vi "Goal Angle Calculation.vi"(5 "Target-Goal X Translation(trans)":dbl, 7 "Target Distance (v)":dbl, 11 "Field-Rel Tgt Angle (theta)":dbl format="%#_13g") -> (1 "Goal Distance (r)":dbl, 3 "Goal Angle (phi)":dbl)   [LabVIEW 2013]
panel:
  out "Vis Tgt - Perp Point Distance (dv)":dbl
  out "Perp. Distance (h)":dbl
  out "Goal - Perp Point Distance (dg)":dbl
  # "d = dg + dv"
  # "goal"
  # "vision target"
  # "dg"
  # "dv"
  # "h"
  # "v"
  # "r"
  # "theta"
  # "phi"
  # "cam angle + servo angle + gyro angle"
  # "robot"
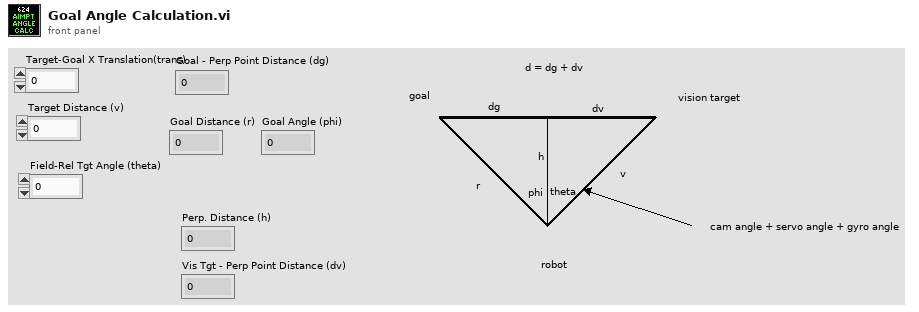
[diagram p1: front panel]
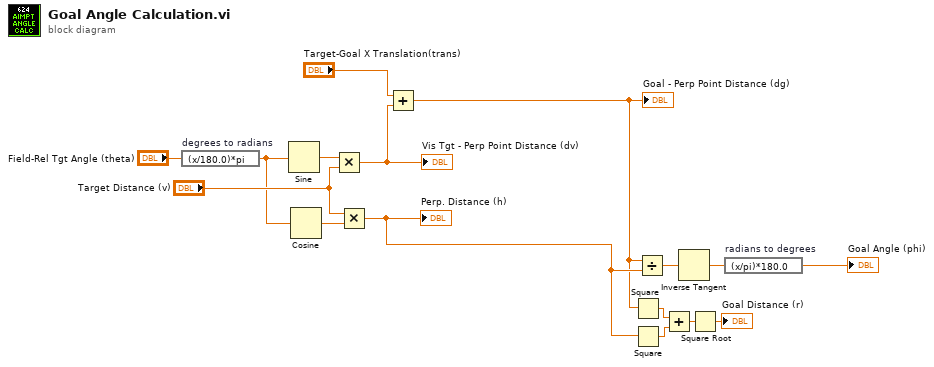
[diagram p0: block diagram]
diagram:
  n1 = expression code="(x/180.0)*pi" "degrees to radians"("Field-Rel Tgt Angle (theta)") -> (w4:dbl)
  n2 = Sine(x=w4) -> (sin(x)=w16:dbl)
  n3 = Cosine(x=w4) -> (cos(x)=w14:dbl)
  n4 = Multiply(x=w16, y="Target Distance (v)") -> (x*y=w6:dbl)
  "Vis Tgt - Perp Point Distance (dv)" <- w6
  n5 = Multiply(x="Target Distance (v)", y=w14) -> (x*y=w7:dbl)
  "Perp. Distance (h)" <- w7
  n6 = Add(x="Target-Goal X Translation(trans)", y=w6) -> (x+y=w5:dbl)
  "Goal - Perp Point Distance (dg)" <- w5
  n7 = Square(x=w5) -> (x^2=w10:dbl)
  n8 = Square(x=w7) -> (x^2=w11:dbl)
  n9 = Divide(x=w5, y=w7) -> (x/y=w15:dbl)
  n10 = Add(x=w10, y=w11) -> (x+y=w9:dbl)
  n11 = Inverse Tangent(1:w15) -> (0:w2:dbl)
  n12 = Square Root(x=w9) -> (sqrt(x)=→"Goal Distance (r)":dbl)
  n13 = expression code="(x/pi)*180.0" "radians to degrees"(w2) -> (→"Goal Angle (phi)":dbl)
